vi "Convert to Absolute Path.vi"(8 "error in":errorcluster, 11 "path":path) -> (0 "error out":errorcluster, 3 "absolute path":path)   [LabVIEW 2019]
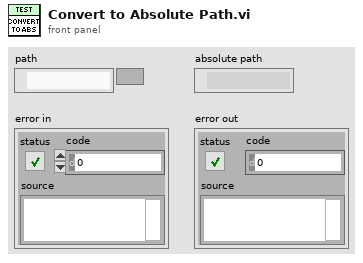
[diagram p1: front panel]
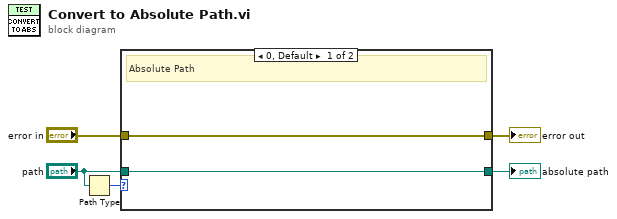
[diagram p0: block diagram]
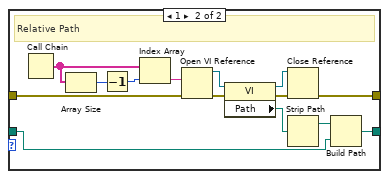
[diagram p2: hidden frame]
diagram:
  n1 = Path Type(1:"path") -> (0:w4:i16)
  n2 = case shown="0, Default" w4 {
    tunnel: [w7 w11] -> w3
    tunnel: "path" -> [w7 w10]
    tunnel: "error in" -> [w6 w9]
    tunnel: [w6 w8] -> w1
    frame 0, Default {
      # "Absolute Path"
    }
    frame 1 {
      # "Relative Path"
      n3 = Call Chain() -> (call chain=w19:string[])
      n4 = Array Size(array=w19) -> (size(s)=w21:i32)
      n5 = Decrement(x=w21) -> (x-1=w20:i32)
      n6 = Index Array(array=w19, index=w20) -> (element=w18:string)
      n7 = Open VI Reference(vi path=w18, error in (no error)=w9) -> (vi reference=w17:refnum<vi>, error out=w16:errorcluster)  [unwired: 4 in]
      n8 = property class="VI"(reference=w17, error in=w16) -> (reference out=w14:refnum<vi>, error out=w15:errorcluster, "Path"=w13:path)
      n9 = Close Reference(reference=w14, error in (no error)=w15) -> (error out=w8:errorcluster)
      n10 = Strip Path(path=w13) -> (stripped path=w12:path)  [unwired: 1 out]
      n11 = Build Path(base path=w12, name or relative path=w10) -> (appended path=w11:path)
    }
  }
  "absolute path" <- w3
  "error out" <- w1
